vi "Activity_5.vi"() -> ()   [LabVIEW 2015]
panel:
  in  "stop":bool
  in  "Tab Control":T1(tab)=enum."Punto Flotante"
  in  "8 Bits":u8=255
  out "8 Bits":u8=255
  in  "16 Bits":u16=65535
  out "16 Bits":u16=65535
  in  "32 Bits":u32=4294967295
  out "32 Bits":u32=4294967295
  in  "64 Bits":u64=18446744073709551615
  out "64 Bits":u64=18446744073709551615
  in  "64 Bits":i64=9223372036854775807
  in  "32 Bits":i32=2147483647
  in  "16 Bits":i16=32767
  in  "8 Bits":i8=127
  out "8 Bits":i8=127
  out "16 Bits":i16=32767
  out "32 Bits":i32=2147483647
  out "64 Bits":i64=9223372036854775807
  in  "Punto Flotante\nPrecision Extendida":dbl
  in  "Punto Flotante\nDoble precisión":dbl
  in  "Punto Flotante\nPrecisión Simple":sgl format="%#_6f"
  out "Punto Flotante\nPrecisión Simple":sgl format="%#_6f"
  out "Punto Flotante\nDoble precisión 2":dbl
  out "Punto Flotante\nPrecision Extendida 2":dbl
  in  "Punto Flotante Complejo\nPrecision Extendida":cxt format="%#_6f"
  in  "Punto Flotante Complejo\nPrecisión Doble":cdb format="%#_6f"
  in  "Punto Flotante Complejo\nPrecisión Simple":csg format="%#_6f"
  out "Punto Flotante Complejo\nPrecisión Simple":csg format="%#_6f"
  out "Punto Flotante Complejo\nPrecisión Doble 2":cdb format="%#_6f"
  out "Punto Flotante Complejo\nPrecision Extendida 2":cxt format="%#_6f"
  # "Fecha de Entrega: 9/2/2019"
  # "Tipos de Datos"
  # "Serrano Bermúdez Luis Esteban"
  # "Descripción:"
  # "Muestra los ndiferentes tipos de datos que se usan en\nLabView distribuidos en diferentes pestañas"
  # "Números Enteros sin Signo"
  # "Números Enteros con Signo"
  # "Punto Flotante"
  # "Punto Flotante Complejos"
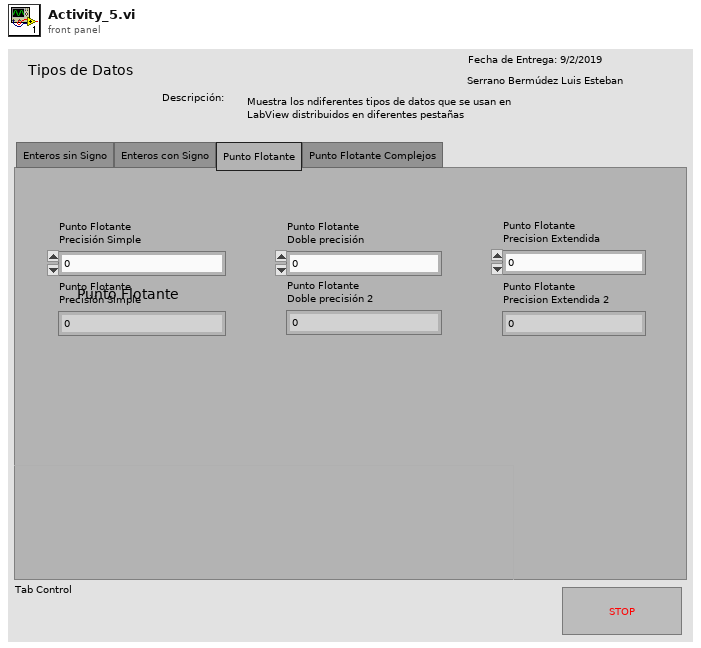
[diagram p1: front panel]
types:
  T1 = enum32{"Enteros sin Signo", "Enteros con Signo", "Punto Flotante", "Punto Flotante Complejos"}
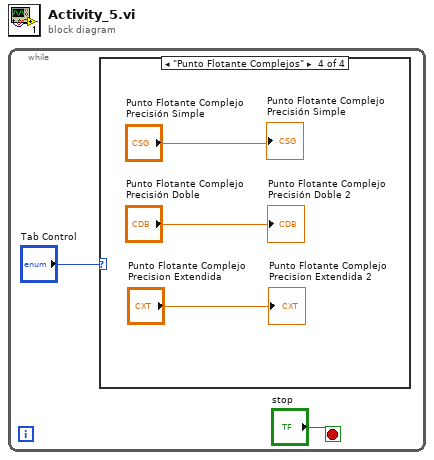
[diagram p0: block diagram]
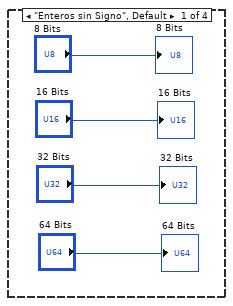
[diagram p2: hidden frame]
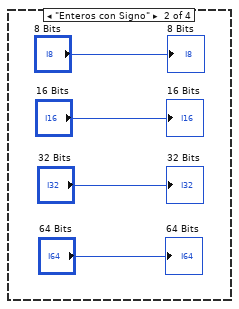
[diagram p3: hidden frame]
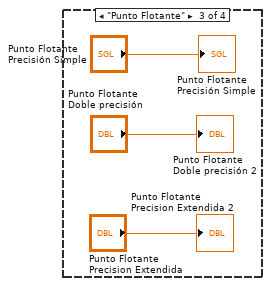
[diagram p4: hidden frame]
diagram:
  n1 = while {
    stop <- "stop" stop-if-true
    n2 = case shown="\"Punto Flotante Complejos\"" "Tab Control" {
      frame "Enteros sin Signo", Default {
        "8 Bits" <- "8 Bits"
        "16 Bits" <- "16 Bits"
        "32 Bits" <- "32 Bits"
        "64 Bits" <- "64 Bits"
      }
      frame "Enteros con Signo" {
        "8 Bits" <- "8 Bits"
        "16 Bits" <- "16 Bits"
        "32 Bits" <- "32 Bits"
        "64 Bits" <- "64 Bits"
      }
      frame "Punto Flotante" {
        "Punto Flotante\nPrecisión Simple" <- "Punto Flotante\nPrecisión Simple"
        "Punto Flotante\nDoble precisión 2" <- "Punto Flotante\nDoble precisión"
        "Punto Flotante\nPrecision Extendida 2" <- "Punto Flotante\nPrecision Extendida"
      }
      frame "Punto Flotante Complejos" {
        "Punto Flotante Complejo\nPrecisión Simple" <- "Punto Flotante Complejo\nPrecisión Simple"
        "Punto Flotante Complejo\nPrecisión Doble 2" <- "Punto Flotante Complejo\nPrecisión Doble"
        "Punto Flotante Complejo\nPrecision Extendida 2" <- "Punto Flotante Complejo\nPrecision Extendida"
      }
    }
  }
